vi "SeCrTs-TC waveform Samples bulider .vi"(7 "Samples":i32=10, 8 "Data FIFO Ref":T1, 9 "Data input":waveform(dbl)[](array[waveform]), 10 "Data_init":dbl[][](array[numeric]), 11 "Waveform_Init":timestamp[][](array[timestamp])) -> (1 "Data out":waveform(dbl)[](array[waveform]), 2 "Data_SR":dbl[][](array[numeric]), 3 "WF_SR":timestamp[][](array[timestamp]))   [LabVIEW 2022 SP3]
uses:
  RT Controls/Data FIFO.ctl
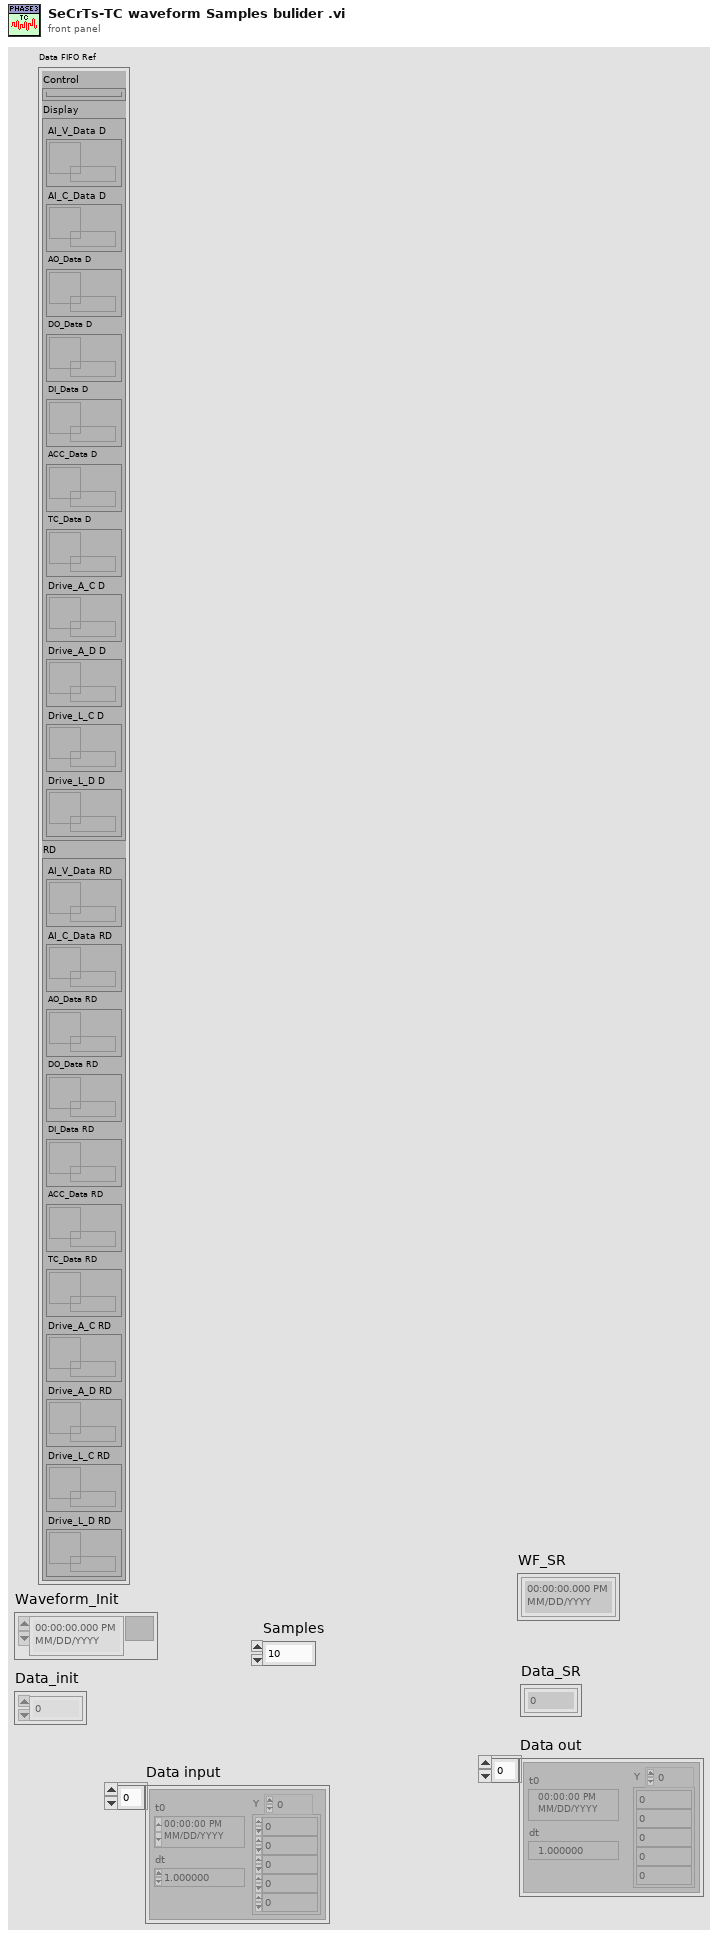
[diagram p1: front panel]
types:
  T1 = typedef "Data FIFO.ctl" = cluster{"Control":cluster{"AI_V_Data":refnum<queue>, "AI_C_Data":refnum<queue>, "AO_Data":refnum<queue>, "DO_Data":refnum<queue>, "DI_Data":refnum<queue>, "ACC_Data":refnum<queue>, "TC_Data":refnum<queue>, "Drive_A_C":refnum<queue>, "Drive_A_D":refnum<queue>, "Drive_L_C":refnum<queue>, "Drive_L_D":refnum<queue>}, "Display":cluster{"AI_V_Data D":refnum<queue>, "AI_C_Data D":refnum<queue>, "AO_Data D":refnum<queue>, "DO_Data D":refnum<queue>, "DI_Data D":refnum<queue>, "ACC_Data D":refnum<queue>, "TC_Data D":refnum<queue>, "Drive_A_C D":refnum<queue>, "Drive_A_D D":refnum<queue>, "Drive_L_C D":refnum<queue>, "Drive_L_D D":refnum<queue>}, "RD":cluster{"AI_V_Data RD":refnum<queue>, "AI_C_Data RD":refnum<queue>, "AO_Data RD":refnum<queue>, "DO_Data RD":refnum<queue>, "DI_Data RD":refnum<queue>, "ACC_Data RD":refnum<queue>, "TC_Data RD":refnum<queue>, "Drive_A_C RD":refnum<queue>, "Drive_A_D RD":refnum<queue>, "Drive_L_C RD":refnum<queue>, "Drive_L_D RD":refnum<queue>}}
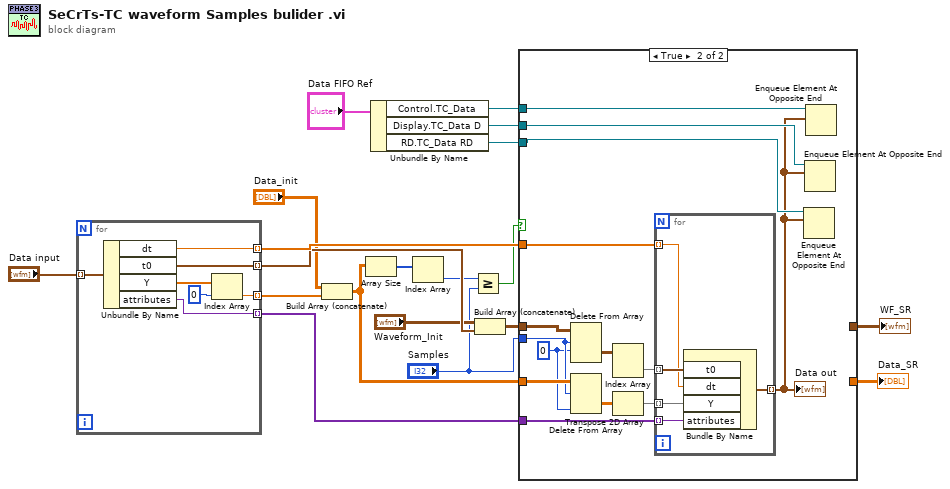
[diagram p0: block diagram]
diagram:
  n1 = for {
    tunnel: "Data input" -> [w26] mode=indexing
    tunnel: [w24] -> w7 mode=indexing
    tunnel: [w22] -> w15 mode=indexing
    tunnel: [w21] -> w18 mode=indexing
    tunnel: [w20] -> w19 mode=indexing
    n2 = Unbundle By Name(w26) -> ("dt"=w20:dbl, "t0"=w22:timestamp, "Y"=w25:dbl[], "attributes"=w21:variant)
    n3 = Index Array(array=w25, index=0) -> (element=w24:dbl)
  }
  n4 = Build Array (concatenate)("Data_init", w7) -> (w10:dbl[][])
  n5 = Array Size(array=w10) -> (size(s)=w8:i32[])
  n6 = Unbundle By Name("Data FIFO Ref") -> ("Control.TC_Data"=w3:refnum<queue>, "Display.TC_Data D"=w2:refnum<queue>, "RD.TC_Data RD"=w1:refnum<queue>)
  n7 = Index Array(array=w8) -> (element=w9:i32)  [unwired: 1 in]
  n8 = Greater Or Equal?(x=w9, y="Samples") -> (x >= y?=w12:bool)
  n9 = Build Array (concatenate)("Waveform_Init", w15) -> (w16:timestamp[][])
  n10 = case shown="True" w12 {
    tunnel: w10 -> [w28 w42]
    tunnel: [w28 _] -> w11
    tunnel: w16 -> [w27 w40]
    tunnel: [w27 _] -> w17
    tunnel: w18 -> [_ w37]
    tunnel: w19 -> [_ w35]
    tunnel: "Samples" -> [_ w34]
    tunnel: w3 -> [_ w32]
    tunnel: w2 -> [_ w31]
    tunnel: w1 -> [_ w30]
    frame False {
    }
    frame True {
      w33 = 0 ("index (row)")
      n11 = Delete From Array(array=w40, length=w34, index (row)=w33) -> (deleted portion=w39:timestamp[][])  [unwired: 1 in, 1 out]
      n12 = Delete From Array(array=w42, length=w34, index (col)=w33) -> (deleted portion=w41:dbl[][])  [unwired: 1 in, 1 out]
      n13 = Index Array(array=w39) -> (element=w38:timestamp[])  [unwired: 2 in]
      n14 = Transpose 2D Array(2D array=w41) -> (transposed array=w36:dbl[][])
      n15 = for {
        tunnel: w36 -> [w47] mode=indexing
        tunnel: w38 -> [w46] mode=indexing
        tunnel: w37 -> [w45] mode=indexing
        tunnel: [w44] -> w29 mode=indexing
        tunnel: w35 -> [w43] mode=indexing
        n16 = Bundle By Name("t0"=w46, "dt"=w43, "Y"=w47, "attributes"=w45) -> (w44:waveform(dbl))  [unwired: 1 in]
      }
      "Data out" <- w29
      n17 = Enqueue Element At Opposite End(queue=w30, element=w29) -> ()  [unwired: 2 in, 3 out]
      n18 = Enqueue Element At Opposite End(queue=w31, element=w29) -> ()  [unwired: 2 in, 3 out]
      n19 = Enqueue Element At Opposite End(queue=w32, element=w29) -> ()  [unwired: 2 in, 3 out]
    }
  }
  "WF_SR" <- w17
  "Data_SR" <- w11
